vi "Send Change Page.vi"(7 "Message Priority (Normal)":T2=enum."Normal", 8 "error in (no error)":errorcluster, 10 "Service State":T1(ring)=enum."HouseKeeping", 11 "Message Enqueuer":refnum<class "Message Enqueuer.lvclass">) -> (0 "error out":errorcluster, 3 "Message Enqueuer out":refnum<class "Message Enqueuer.lvclass">)   [LabVIEW 2023, in "Room Service Manager UI.lvlib" / "Change Page Msg.lvclass"]
doc: "This VI sends the message to an actor."
uses:
  Change Page Msg.lvclass
  <vilib>/ActorFramework/Message Enqueuer/Message Enqueuer.lvclass
  <vilib>/ActorFramework/Message Enqueuer/Message Priority.ctl
  C:/Program Files/National Instruments/LabVIEW 2023/vi.lib/ActorFramework/Message/Message.lvclass
  Change Page Msg.lvclass/Change Page Msg.ctl
  <vilib>/ActorFramework/Message Enqueuer/Message Enqueuer.lvclass/Message Enqueuer.ctl
  <vilib>/ActorFramework/Message Priority Queue/Priority Enqueue.vi
  C:/Users/bhaghyaraj/Trainings/NI Actor Framework/SDLC/Room Service Manager UI/Room Service Manager UI Messages/Change Page Msg/Change Page Msg.lvclass
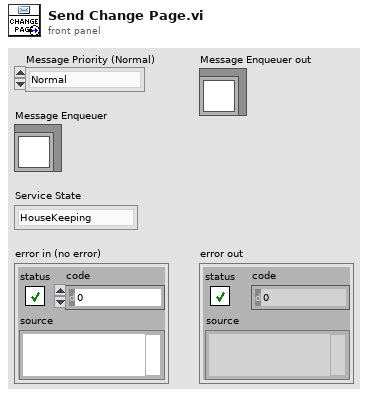
[diagram p1: front panel]
types:
  T1 = enum32{"Home", "HouseKeeping", "Food Order", "Other Request"}
  T2 = typedef "Actor Framework.lvlib/Message Enqueuer.lvclass/Message Priority.ctl" = enum16{"Low", "Normal", "High"}
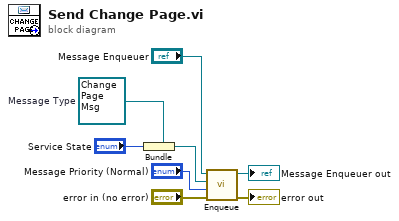
[diagram p0: block diagram]
diagram:
  w5 = refnum<class "Change Page Msg.lvclass"> refnum  # Message Type
  n1 = Bundle(cluster=w5, "Service State") -> (w4:refnum<class "Change Page Msg.lvclass">)
  n2 = call <vilib>:"Enqueue.vi"("error in (no error)"="error in (no error)", "Message Priority (Normal)"="Message Priority (Normal)", "Message"=w4, "Message Enqueuer in"="Message Enqueuer") -> ("error out"=→"error out":errorcluster, "Message Enqueuer in"=→"Message Enqueuer out":refnum<class "Message Enqueuer.lvclass">)  [unwired: 6 in]
